vi "Tree Test.vi"() -> ()   [LabVIEW 2023]
uses:
  SubVIs/Decompose VI (Path).vi
  Support Files/VILab/Classes/Attribute/Attribute.lvclass
  Support Files/VILab/Classes/Data Item/Data Item.lvclass
  Support Files/VILab/Classes/Tree Manager/Tree Manager.lvclass
  VILab.lvlib
panel:
  in  "Rebuild":bool
  in  "Rebuilt":string(tree)
  in  "Tree":string(tree)
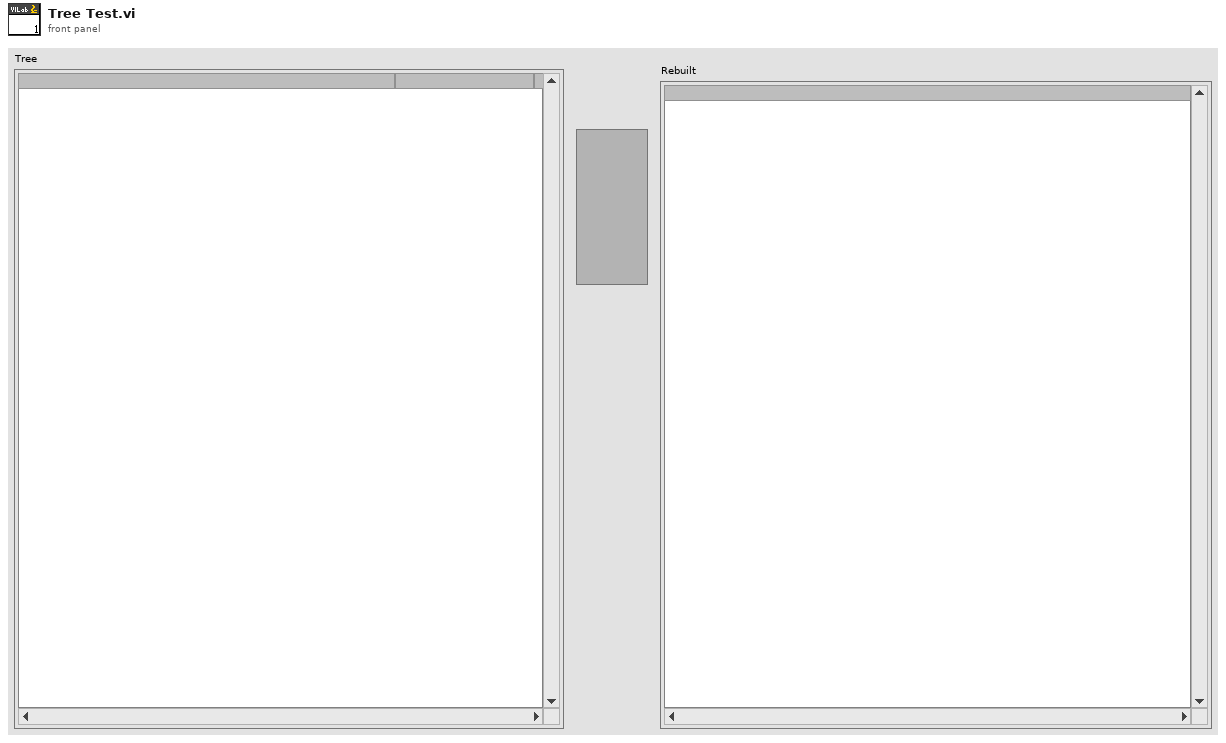
[diagram p1: front panel]
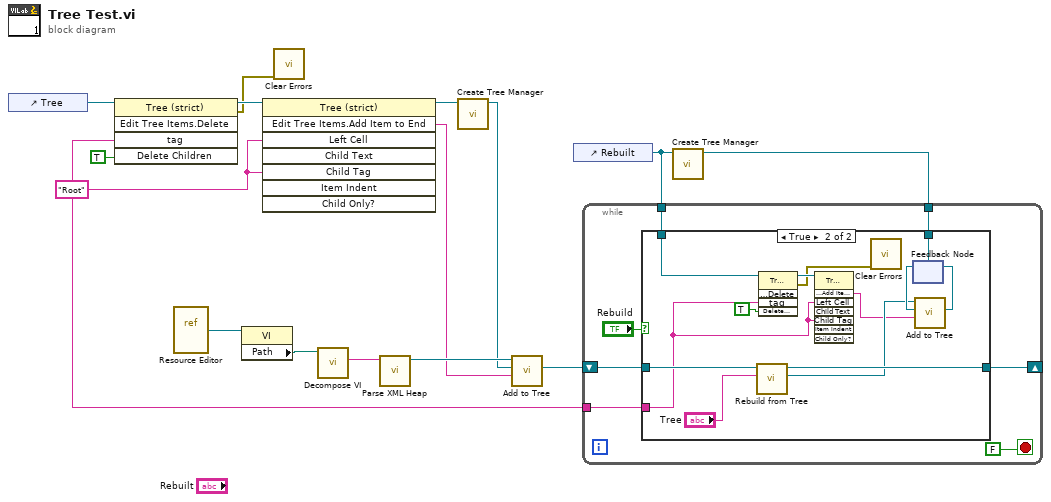
[diagram p0: block diagram]
diagram:
  w7 = "Root"
  n1 = control-ref of="Tree"() -> (w14:refnum<vi>)
  n2 = invoke class="Tree (strict)" method="Edit Tree Items.Delete"(reference=w14, "tag"=w7, "Delete Children"=TRUE ("Delete Children?")) -> (reference out=w12:refnum<vi>, error out=w4:errorcluster)  [unwired: 2 in, 3 out]
  n3 = vi-ref "Resource Editor.vi"() -> (w2:refnum<vi>)
  n4 = property class="VI"(reference=w2) -> ("Path"=w15:path)  [unwired: 1 in, 2 out]
  n5 = invoke class="Tree (strict)" method="Edit Tree Items.Add Item to End"(reference=w12, "Left Cell"=w7, "Child Tag"=w7) -> (reference out=w11:refnum<vi>, "Edit Tree Items:Add Item to End"=w1:string)  [unwired: 5 in, 6 out]
  n6 = call <vilib>:"Clear Errors.vi"("error in (no error)"=w4) -> ()  [unwired: 5 in, 2 out]
  n7 = call-poly "Decompose VI.vi"("VI path"=w15) -> ("Front Panel XML"=w3:string)  [unwired: 6 in, 4 out]
  n8 = call "Parse XML Heap.vi"("XML"=w3) -> ("Root Element"=w10:refnum<class "Attribute.lvclass">)  [unwired: 9 in, 1 out]
  n9 = call "Create Tree Manager.vi"("Tree Control"=w11) -> ("Tree Manager"=w9:refnum<class "Tree Manager.lvclass">)  [unwired: 9 in, 1 out]
  n10 = call-dynamic "Add to Tree.vi"("Parent Tag"=w1, "Tree Manager in"=w9, "Attribute in"=w10) -> ("Tree Manager out"=w8:refnum<class "Tree Manager.lvclass">)  [unwired: 6 in, 2 out]
  n11 = control-ref of="Rebuilt"() -> (w5:refnum<vi>)
  n12 = call "Create Tree Manager.vi"("Tree Control"=w5) -> ("Tree Manager"=w6:refnum<class "Tree Manager.lvclass">)  [unwired: 9 in, 1 out]
  n13 = while {
    tunnel: w7 -> [w21]
    shift-right: [w19] -> _
    shift-left: w8 -> [w22]
    tunnel: w6 -> [w18]
    tunnel: w5 -> [w17]
    stop <- FALSE stop-if-true
    n14 = case shown="True" "Rebuild" {
      tunnel: w22 -> [w23 w36]
      tunnel: w21 -> [_ w27]
      tunnel: [w23 w35] -> w19
      tunnel: w18 -> [_ w31]
      tunnel: w17 -> [_ w32]
      frame False {
      }
      frame True {
        n15 = call "Rebuild from Tree.vi"("Tag"="Tree", "Tree Manager in"=w36) -> ("Rebuilt Item"=w28:refnum<class "Data Item.lvclass">, "Tree Manager out"=w35:refnum<class "Tree Manager.lvclass">)  [unwired: 7 in, 1 out]
        n16 = invoke class="Tree (strict)" method="Edit Tree Items.Delete"(reference=w32, "tag"=w27, "Delete Children"=TRUE ("Delete Children?")) -> (reference out=w34:refnum<vi>, error out=w26:errorcluster)  [unwired: 2 in, 3 out]
        n17 = invoke class="Tree (strict)" method="Edit Tree Items.Add Item to End"(reference=w34, "Left Cell"=w27, "Child Tag"=w27) -> ("Edit Tree Items:Add Item to End"=w24:string)  [unwired: 5 in, 7 out]
        n18 = call <vilib>:"Clear Errors.vi"("error in (no error)"=w26) -> ()  [unwired: 5 in, 2 out]
        n19 = feedback #1(w31) -> (w30:refnum<class "Tree Manager.lvclass">)
        n20 = call-dynamic "Add to Tree.vi"("Parent Tag"=w24, "Tree Manager in"=w30, "Data Item in"=w28) -> ("Tree Manager out"=w29:refnum<class "Tree Manager.lvclass">)  [unwired: 6 in, 2 out]
        n21 = feedback-in #1(w29) -> ()
      }
    }
  }
